vi "Get Sensor Previous Button Visibility.vi"(8 "error in (no error)":errorcluster, 11 "Abstract Sensor Previous Button Visibility Msg in":refnum<class "Abstract Sensor Previous Button Visibility Msg.lvclass">) -> (0 "error out":errorcluster, 2 "Sensor Previous Button Visibility":bool, 3 "Abstract Sensor Previous Button Visibility Msg out":refnum<class "Abstract Sensor Previous Button Visibility Msg.lvclass">)   [LabVIEW 2013, in "Sensor Model.lvlib" / "Abstract Sensor Previous Button Visibility Msg.lvclass"]
uses:
  Abstract Sensor Previous Button Visibility Msg.lvclass
  Abstract Sensor Previous Button Visibility Msg.lvclass/Abstract Sensor Previous Button Visibility Msg.ctl
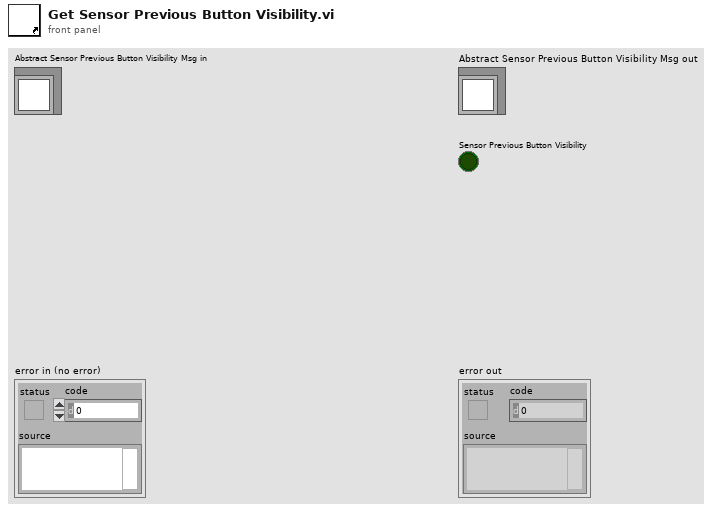
[diagram p1: front panel]
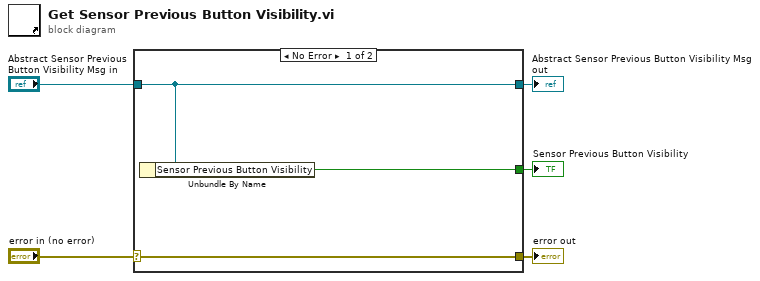
[diagram p0: block diagram]
diagram:
  n1 = case shown="No Error" "error in (no error)" {
    selector: "error in (no error)" -> [w8 w9]
    tunnel: [w8 w9] -> w4
    tunnel: [w7 w10] -> w2
    tunnel: "Abstract Sensor Previous Button Visibility Msg in" -> [w7 w10]
    tunnel: [w6 _] -> w1
    frame No Error {
      n2 = Unbundle By Name(w7) -> ("Sensor Previous Button Visibility"=w6:bool)
    }
    frame Error {
    }
  }
  "error out" <- w4
  "Abstract Sensor Previous Button Visibility Msg out" <- w2
  "Sensor Previous Button Visibility" <- w1
